vi "qetest.vi"() -> ()   [LabVIEW 2017]
panel:
  in  "Boolean":bool
  out "code":i32
  out "description":string
  out "Dll Error Code":u32
  out "error out 2":errorcluster
  out "Max Value":sgl
  out "error out":errorcluster
  out "model":string
  out "QE":i32
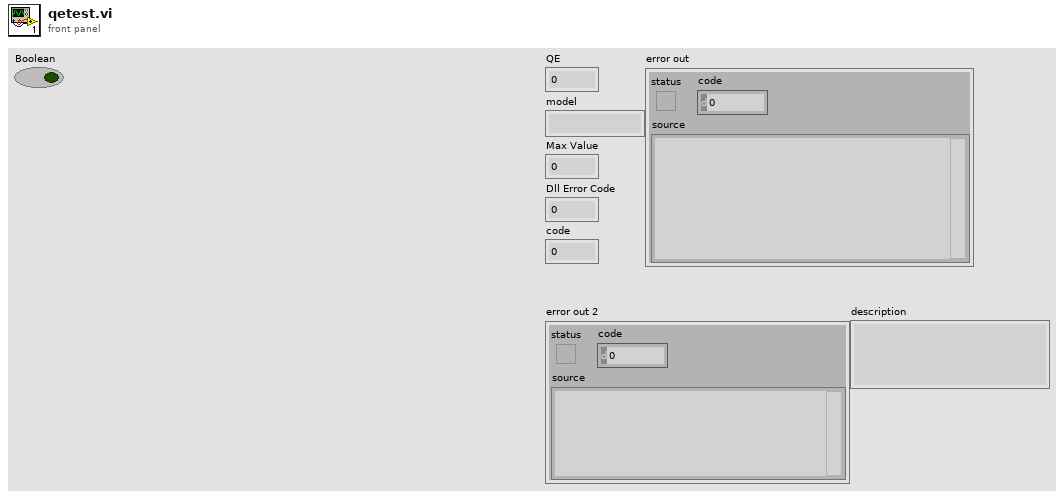
[diagram p1: front panel]
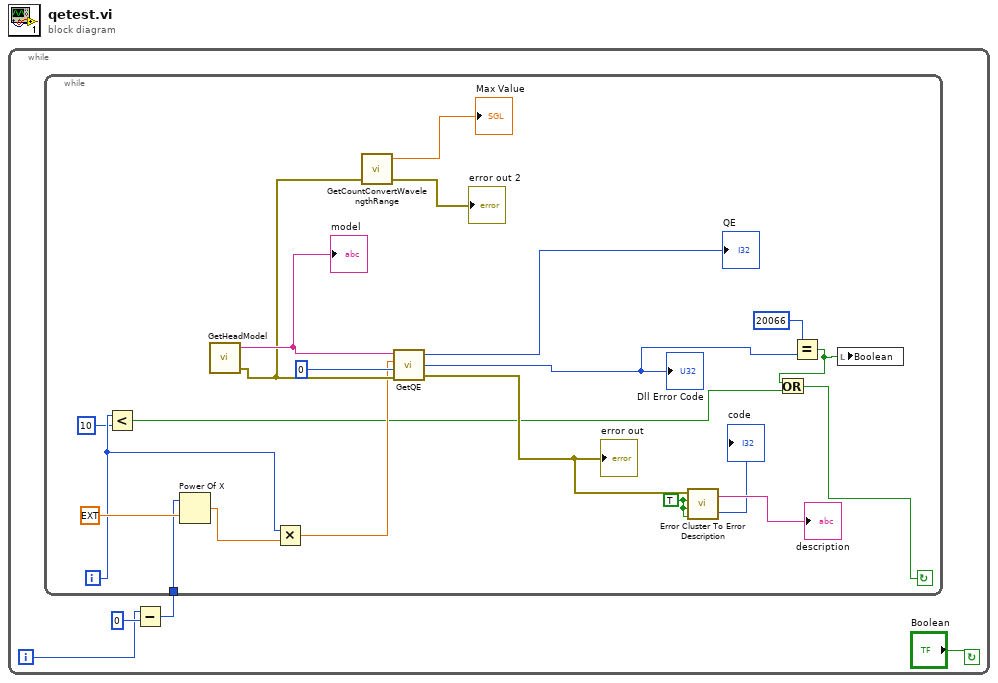
[diagram p0: block diagram]
diagram:
  n1 = while {
    i -> [w3]
    stop <- "Boolean" continue-if-true
    n2 = Subtract(x=w3, y=0) -> (x-y=w1:i32)
    n3 = while {
      tunnel: w1 -> [w8]
      i -> [w7]
      stop <- w10 continue-if-true
      w18 = TRUE ("show name (F)")
      n4 = Less?(x=w7, y=10) -> (x < y?=w5:bool)
      n5 = Power Of X(1:ext 10.0 ("y"), 2:w8) -> (0:w15:ext)
      n6 = call <userlib>:"GetHeadModel.vi"() -> ("error out"=w20:errorcluster, "model"=w25:string)  [unwired: 3 in, 1 out]
      "model" <- w25
      n7 = Multiply(x=w7, y=w15) -> (x*y=w11:ext)
      n8 = call <userlib>:"GetCountConvertWavelengthRange.vi"("error in (no error)"=w20) -> ("error out"=→"error out 2":errorcluster, "Max Value"=→"Max Value":sgl)  [unwired: 2 in, 1 out]
      n9 = call <userlib>:"GetQE.vi"("error in (no error)"=w20, "mode"=u32 0, "wavelength"=w11, "Sensor"=w25) -> ("error out"=w14:errorcluster, "Dll Error Code"=w12:u32, "QE"=→"QE":i32)
      "error out" <- w14
      "Dll Error Code" <- w12
      n10 = call <userlib>:"Error Cluster To Error Description.vi"("show description (T)"=w18, "show DLL error code (F)"=w18, "show name (F)"=w18, "error cluster"=w14) -> ("code"=→"code":i32, "description"=→"description":string)
      n11 = Equal?(x=20066, y=w12) -> (x = y?=w9:bool)
      n12 = Or(x=w9, y=w5) -> (x .or. y?=w10:bool)
      n13 = local write "Boolean"(w9) -> ()
    }
  }
